vi "Write U64.vi"(8 "error in (no error)":errorcluster, 10 "U64":u64, 11 "Event in":refnum<class "Event U64.lvclass">) -> (0 "error out":errorcluster, 3 "Event out":refnum<class "Event U64.lvclass">)   [LabVIEW 2017, in "Event Actors.lvlib" / "Event U64.lvclass"]
uses:
  Event U64.lvclass
  Event U64.lvclass/Event U64.ctl
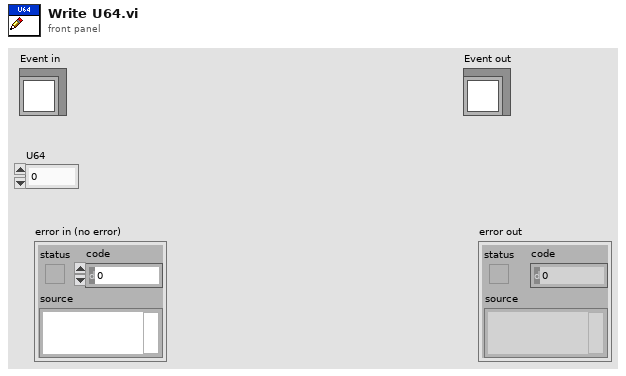
[diagram p1: front panel]
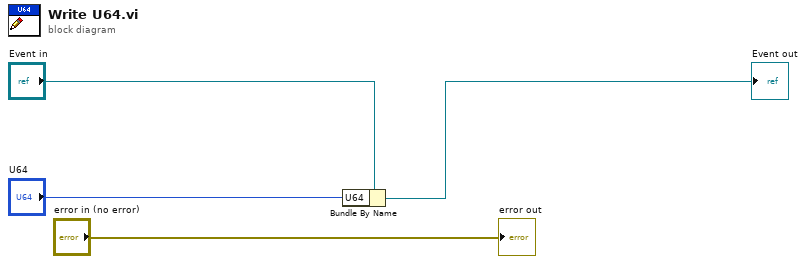
[diagram p0: block diagram]
diagram:
  n1 = Bundle By Name(cluster="Event in", "U64"="U64") -> (→"Event out":refnum<class "Event U64.lvclass">)
  "error out" <- "error in (no error)"
